vi "ORS_ComputePixmapSize8.vi"(9 "height":i16, 10 "width":i16) -> (3 "image data size":i32)   [LabVIEW 2014]
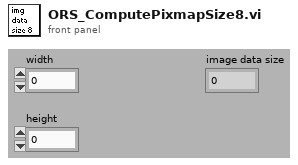
[diagram p1: front panel]
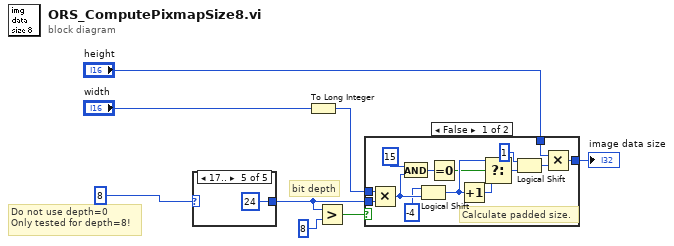
[diagram p0: block diagram]
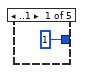
[diagram p2: hidden frame]
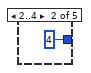
[diagram p3: hidden frame]
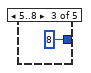
[diagram p4: hidden frame]
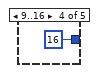
[diagram p5: hidden frame]
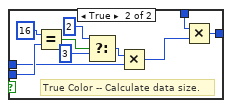
[diagram p6: hidden frame]
diagram:
  # "Do not use depth=0\nOnly tested for depth=8!"
  # "bit depth"
  n1 = case shown="17.." 8 ("image depth") {
    tunnel: [1 4 8 16 24] -> w6
    frame ..1 {
    }
    frame 2..4 {
    }
    frame 5..8 {
    }
    frame 9..16 {
    }
    frame 17.. {
    }
  }
  n2 = To Long Integer(number="width") -> (32bit integer=w5:i32)
  n3 = Greater?(x=w6, y=u8 8) -> (0:w7:bool)
  n4 = case shown="False" w7 {
    tunnel: [w27 w37] -> w1
    tunnel: "height" -> [w23 w36]
    tunnel: w6 -> [w15 w34]
    tunnel: w5 -> [w14 w32]
    frame False {
      # "Calculate padded size."
      n5 = Multiply(x=w14, y=w15) -> (x*y=w17:i32)
      n6 = And(x=15, y=w17) -> (x .and. y?=w19:i32)
      n7 = Logical Shift(y=-4, x=w17) -> (x << y=w21:i32)
      n8 = Equal To 0?(x=w19) -> (x = 0?=w20:bool)
      n9 = Increment(x=w21) -> (x+1=w22:i32)
      n10 = Select(t=w21, s=w20, f=w22) -> (s? t:f=w25:i32)
      n11 = Logical Shift(y=1, x=w25) -> (x << y=w26:i32)
      n12 = Multiply(x=w23, y=w26) -> (x*y=w27:i32)
    }
    frame True {
      # "True Color -- Calculate data size."
      n13 = Equal?(x=16, y=w34) -> (x = y?=w31:bool)
      n14 = Select(t=2, s=w31, f=3) -> (s? t:f=w28:i32)
      n15 = Multiply(x=w28, y=w32) -> (x*y=w35:i32)
      n16 = Multiply(x=w36, y=w35) -> (x*y=w37:i32)
    }
  }
  "image data size" <- w1
